vi "GetProbePlanCoordinates.vi"(8 "Use index as X coord":bool=TRUE, 9 "Probe Card Channels":i32=1) -> (0 "file path":string, 2 "OK?":bool, 3 "Array":T1(array[cluster]))   [LabVIEW 2018] (continued)
616", "Coord On/Off"=TRUE}, {"X"=617.0, "Y"=0.0, "Label"="Strip\t617", "Coord On/Off"=TRUE}, {"X"=618.0, "Y"=0.0, "Label"="Strip\t618", "Coord On/Off"=TRUE}, {"X"=619.0, "Y"=0.0, "Label"="Strip\t619", "Coord On/Off"=TRUE}, {"X"=620.0, "Y"=0.0, "Label"="Strip\t620", "Coord On/Off"=TRUE}, {"X"=621.0, "Y"=0.0, "Label"="Strip\t621", "Coord On/Off"=TRUE}, {"X"=622.0, "Y"=0.0, "Label"="Strip\t622", "Coord On/Off"=TRUE}, {"X"=623.0, "Y"=0.0, "Label"="Strip\t623", "Coord On/Off"=TRUE}, {"X"=624.0, "Y"=0.0, "Label"="Strip\t624", "Coord On/Off"=TRUE}, {"X"=625.0, "Y"=0.0, "Label"="Strip\t625", "Coord On/Off"=TRUE}, {"X"=626.0, "Y"=0.0, "Label"="Strip\t626", "Coord On/Off"=TRUE}, {"X"=627.0, "Y"=0.0, "Label"="Strip\t627", "Coord On/Off"=TRUE}, {"X"=628.0, "Y"=0.0, "Label"="Strip\t628", "Coord On/Off"=TRUE}, {"X"=629.0, "Y"=0.0, "Label"="Strip\t629", "Coord On/Off"=TRUE}, {"X"=630.0, "Y"=0.0, "Label"="Strip\t630", "Coord On/Off"=TRUE}, {"X"=631.0, "Y"=0.0, "Label"="Strip\t631", "Coord On/Off"=TRUE}, {"X"=632.0, "Y"=0.0, "Label"="Strip\t632", "Coord On/Off"=TRUE}, {"X"=633.0, "Y"=0.0, "Label"="Strip\t633", "Coord On/Off"=TRUE}, {"X"=634.0, "Y"=0.0, "Label"="Strip\t634", "Coord On/Off"=TRUE}, {"X"=635.0, "Y"=0.0, "Label"="Strip\t635", "Coord On/Off"=TRUE}, {"X"=636.0, "Y"=0.0, "Label"="Strip\t636", "Coord On/Off"=TRUE}, {"X"=637.0, "Y"=0.0, "Label"="Strip\t637", "Coord On/Off"=TRUE}, {"X"=638.0, "Y"=0.0, "Label"="Strip\t638", "Coord On/Off"=TRUE}, {"X"=639.0, "Y"=0.0, "Label"="Strip\t639", "Coord On/Off"=TRUE}, {"X"=640.0, "Y"=0.0, "Label"="Strip\t640", "Coord On/Off"=TRUE}, {"X"=641.0, "Y"=0.0, "Label"="Strip\t641", "Coord On/Off"=TRUE}, {"X"=642.0, "Y"=0.0, "Label"="Strip\t642", "Coord On/Off"=TRUE}, {"X"=643.0, "Y"=0.0, "Label"="Strip\t643", "Coord On/Off"=TRUE}, {"X"=644.0, "Y"=0.0, "Label"="Strip\t644", "Coord On/Off"=TRUE}, {"X"=645.0, "Y"=0.0, "Label"="Strip\t645", "Coord On/Off"=TRUE}, {"X"=646.0, "Y"=0.0, "Label"="Strip\t646", "Coord On/Off"=TRUE}, {"X"=647.0, "Y"=0.0, "Label"="Strip\t647", "Coord On/Off"=TRUE}, {"X"=648.0, "Y"=0.0, "Label"="Strip\t648", "Coord On/Off"=TRUE}, {"X"=649.0, "Y"=0.0, "Label"="Strip\t649", "Coord On/Off"=TRUE}, {"X"=650.0, "Y"=0.0, "Label"="Strip\t650", "Coord On/Off"=TRUE}, {"X"=651.0, "Y"=0.0, "Label"="Strip\t651", "Coord On/Off"=TRUE}, {"X"=652.0, "Y"=0.0, "Label"="Strip\t652", "Coord On/Off"=TRUE}, {"X"=653.0, "Y"=0.0, "Label"="Strip\t653", "Coord On/Off"=TRUE}, {"X"=654.0, "Y"=0.0, "Label"="Strip\t654", "Coord On/Off"=TRUE}, {"X"=655.0, "Y"=0.0, "Label"="Strip\t655", "Coord On/Off"=TRUE}, {"X"=656.0, "Y"=0.0, "Label"="Strip\t656", "Coord On/Off"=TRUE}, {"X"=657.0, "Y"=0.0, "Label"="Strip\t657", "Coord On/Off"=TRUE}, {"X"=658.0, "Y"=0.0, "Label"="Strip\t658", "Coord On/Off"=TRUE}, {"X"=659.0, "Y"=0.0, "Label"="Strip\t659", "Coord On/Off"=TRUE}, {"X"=660.0, "Y"=0.0, "Label"="Strip\t660", "Coord On/Off"=TRUE}, {"X"=661.0, "Y"=0.0, "Label"="Strip\t661", "Coord On/Off"=TRUE}, {"X"=662.0, "Y"=0.0, "Label"="Strip\t662", "Coord On/Off"=TRUE}, {"X"=663.0, "Y"=0.0, "Label"="Strip\t663", "Coord On/Off"=TRUE}, {"X"=664.0, "Y"=0.0, "Label"="Strip\t664", "Coord On/Off"=TRUE}, {"X"=665.0, "Y"=0.0, "Label"="Strip\t665", "Coord On/Off"=TRUE}, {"X"=666.0, "Y"=0.0, "Label"="Strip\t666", "Coord On/Off"=TRUE}, {"X"=667.0, "Y"=0.0, "Label"="Strip\t667", "Coord On/Off"=TRUE}, {"X"=668.0, "Y"=0.0, "Label"="Strip\t668", "Coord On/Off"=TRUE}, {"X"=669.0, "Y"=0.0, "Label"="Strip\t669", "Coord On/Off"=TRUE}, {"X"=670.0, "Y"=0.0, "Label"="Strip\t670", "Coord On/Off"=TRUE}, {"X"=671.0, "Y"=0.0, "Label"="Strip\t671", "Coord On/Off"=TRUE}, {"X"=672.0, "Y"=0.0, "Label"="Strip\t672", "Coord On/Off"=TRUE}, {"X"=673.0, "Y"=0.0, "Label"="Strip\t673", "Coord On/Off"=TRUE}, {"X"=674.0, "Y"=0.0, "Label"="Strip\t674", "Coord On/Off"=TRUE}, {"X"=675.0, "Y"=0.0, "Label"="Strip\t675", "Coord On/Off"=TRUE}, {"X"=676.0, "Y"=0.0, "Label"="Strip\t676", "Coord On/Off"=TRUE}, {"X"=677.0, "Y"=0.0, "Label"="Strip\t677", "Coord On/Off"=TRUE}, {"X"=678.0, "Y"=0.0, "Label"="Strip\t678", "Coord On/Off"=TRUE}, {"X"=679.0, "Y"=0.0, "Label"="Strip\t679", "Coord On/Off"=TRUE}, {"X"=680.0, "Y"=0.0, "Label"="Strip\t680", "Coord On/Off"=TRUE}, {"X"=681.0, "Y"=0.0, "Label"="Strip\t681", "Coord On/Off"=TRUE}, {"X"=682.0, "Y"=0.0, "Label"="Strip\t682", "Coord On/Off"=TRUE}, {"X"=683.0, "Y"=0.0, "Label"="Strip\t683", "Coord On/Off"=TRUE}, {"X"=684.0, "Y"=0.0, "Label"="Strip\t684", "Coord On/Off"=TRUE}, {"X"=685.0, "Y"=0.0, "Label"="Strip\t685", "Coord On/Off"=TRUE}, {"X"=686.0, "Y"=0.0, "Label"="Strip\t686", "Coord On/Off"=TRUE}, {"X"=687.0, "Y"=0.0, "Label"="Strip\t687", "Coord On/Off"=TRUE}, {"X"=688.0, "Y"=0.0, "Label"="Strip\t688", "Coord On/Off"=TRUE}, {"X"=689.0, "Y"=0.0, "Label"="Strip\t689", "Coord On/Off"=TRUE}, {"X"=690.0, "Y"=0.0, "Label"="Strip\t690", "Coord On/Off"=TRUE}, {"X"=691.0, "Y"=0.0, "Label"="Strip\t691", "Coord On/Off"=TRUE}, {"X"=692.0, "Y"=0.0, "Label"="Strip\t692", "Coord On/Off"=TRUE}, {"X"=693.0, "Y"=0.0, "Label"="Strip\t693", "Coord On/Off"=TRUE}, {"X"=694.0, "Y"=0.0, "Label"="Strip\t694", "Coord On/Off"=TRUE}, {"X"=695.0, "Y"=0.0, "Label"="Strip\t695", "Coord On/Off"=TRUE}, {"X"=696.0, "Y"=0.0, "Label"="Strip\t696", "Coord On/Off"=TRUE}, {"X"=697.0, "Y"=0.0, "Label"="Strip\t697", "Coord On/Off"=TRUE}, {"X"=698.0, "Y"=0.0, "Label"="Strip\t698", "Coord On/Off"=TRUE}, {"X"=699.0, "Y"=0.0, "Label"="Strip\t699", "Coord On/Off"=TRUE}, {"X"=700.0, "Y"=0.0, "Label"="Strip\t700", "Coord On/Off"=TRUE}, {"X"=701.0, "Y"=0.0, "Label"="Strip\t701", "Coord On/Off"=TRUE}, {"X"=702.0, "Y"=0.0, "Label"="Strip\t702", "Coord On/Off"=TRUE}, {"X"=703.0, "Y"=0.0, "Label"="Strip\t703", "Coord On/Off"=TRUE}, {"X"=704.0, "Y"=0.0, "Label"="Strip\t704", "Coord On/Off"=TRUE}, {"X"=705.0, "Y"=0.0, "Label"="Strip\t705", "Coord On/Off"=TRUE}, {"X"=706.0, "Y"=0.0, "Label"="Strip\t706", "Coord On/Off"=TRUE}, {"X"=707.0, "Y"=0.0, "Label"="Strip\t707", "Coord On/Off"=TRUE}, {"X"=708.0, "Y"=0.0, "Label"="Strip\t708", "Coord On/Off"=TRUE}, {"X"=709.0, "Y"=0.0, "Label"="Strip\t709", "Coord On/Off"=TRUE}, {"X"=710.0, "Y"=0.0, "Label"="Strip\t710", "Coord On/Off"=TRUE}, {"X"=711.0, "Y"=0.0, "Label"="Strip\t711", "Coord On/Off"=TRUE}, {"X"=712.0, "Y"=0.0, "Label"="Strip\t712", "Coord On/Off"=TRUE}, {"X"=713.0, "Y"=0.0, "Label"="Strip\t713", "Coord On/Off"=TRUE}, {"X"=714.0, "Y"=0.0, "Label"="Strip\t714", "Coord On/Off"=TRUE}, {"X"=715.0, "Y"=0.0, "Label"="Strip\t715", "Coord On/Off"=TRUE}, {"X"=716.0, "Y"=0.0, "Label"="Strip\t716", "Coord On/Off"=TRUE}, {"X"=717.0, "Y"=0.0, "Label"="Strip\t717", "Coord On/Off"=TRUE}, {"X"=718.0, "Y"=0.0, "Label"="Strip\t718", "Coord On/Off"=TRUE}, {"X"=719.0, "Y"=0.0, "Label"="Strip\t719", "Coord On/Off"=TRUE}, {"X"=720.0, "Y"=0.0, "Label"="Strip\t720", "Coord On/Off"=TRUE}, {"X"=721.0, "Y"=0.0, "Label"="Strip\t721", "Coord On/Off"=TRUE}, {"X"=722.0, "Y"=0.0, "Label"="Strip\t722", "Coord On/Off"=TRUE}, {"X"=723.0, "Y"=0.0, "Label"="Strip\t723", "Coord On/Off"=TRUE}, {"X"=724.0, "Y"=0.0, "Label"="Strip\t724", "Coord On/Off"=TRUE}, {"X"=725.0, "Y"=0.0, "Label"="Strip\t725", "Coord On/Off"=TRUE}, {"X"=726.0, "Y"=0.0, "Label"="Strip\t726", "Coord On/Off"=TRUE}, {"X"=727.0, "Y"=0.0, "Label"="Strip\t727", "Coord On/Off"=TRUE}, {"X"=728.0, "Y"=0.0, "Label"="Strip\t728", "Coord On/Off"=TRUE}, {"X"=729.0, "Y"=0.0, "Label"="Strip\t729", "Coord On/Off"=TRUE}, {"X"=730.0, "Y"=0.0, "Label"="Strip\t730", "Coord On/Off"=TRUE}, {"X"=731.0, "Y"=0.0, "Label"="Strip\t731", "Coord On/Off"=TRUE}, {"X"=732.0, "Y"=0.0, "Label"="Strip\t732", "Coord On/Off"=TRUE}, {"X"=733.0, "Y"=0.0, "Label"="Strip\t733", "Coord On/Off"=TRUE}, {"X"=734.0, "Y"=0.0, "Label"="Strip\t734", "Coord On/Off"=TRUE}, {"X"=735.0, "Y"=0.0, "Label"="Strip\t735", "Coord On/Off"=TRUE}, {"X"=736.0, "Y"=0.0, "Label"="Strip\t736", "Coord On/Off"=TRUE}, {"X"=737.0, "Y"=0.0, "Label"="Strip\t737", "Coord On/Off"=TRUE}, {"X"=738.0, "Y"=0.0, "Label"="Strip\t738", "Coord On/Off"=TRUE}, {"X"=739.0, "Y"=0.0, "Label"="Strip\t739", "Coord On/Off"=TRUE}, {"X"=740.0, "Y"=0.0, "Label"="Strip\t740", "Coord On/Off"=TRUE}, {"X"=741.0, "Y"=0.0, "Label"="Strip\t741", "Coord On/Off"=TRUE}, {"X"=742.0, "Y"=0.0, "Label"="Strip\t742", "Coord On/Off"=TRUE}, {"X"=743.0, "Y"=0.0, "Label"="Strip\t743", "Coord On/Off"=TRUE}, {"X"=744.0, "Y"=0.0, "Label"="Strip\t744", "Coord On/Off"=TRUE}, {"X"=745.0, "Y"=0.0, "Label"="Strip\t745", "Coord On/Off"=TRUE}, {"X"=746.0, "Y"=0.0, "Label"="Strip\t746", "Coord On/Off"=TRUE}, {"X"=747.0, "Y"=0.0, "Label"="Strip\t747", "Coord On/Off"=TRUE}, {"X"=748.0, "Y"=0.0, "Label"="Strip\t748", "Coord On/Off"=TRUE}, {"X"=749.0, "Y"=0.0, "Label"="Strip\t749", "Coord On/Off"=TRUE}, {"X"=750.0, "Y"=0.0, "Label"="Strip\t750", "Coord On/Off"=TRUE}, {"X"=751.0, "Y"=0.0, "Label"="Strip\t751", "Coord On/Off"=TRUE}, {"X"=752.0, "Y"=0.0, "Label"="Strip\t752", "Coord On/Off"=TRUE}, {"X"=753.0, "Y"=0.0, "Label"="Strip\t753", "Coord On/Off"=TRUE}, {"X"=754.0, "Y"=0.0, "Label"="Strip\t754", "Coord On/Off"=TRUE}, {"X"=755.0, "Y"=0.0, "Label"="Strip\t755", "Coord On/Off"=TRUE}, {"X"=756.0, "Y"=0.0, "Label"="Strip\t756", "Coord On/Off"=TRUE}, {"X"=757.0, "Y"=0.0, "Label"="Strip\t757", "Coord On/Off"=TRUE}, {"X"=758.0, "Y"=0.0, "Label"="Strip\t758", "Coord On/Off"=TRUE}, {"X"=759.0, "Y"=0.0, "Label"="Strip\t759", "Coord On/Off"=TRUE}, {"X"=760.0, "Y"=0.0, "Label"="Strip\t760", "Coord On/Off"=TRUE}, {"X"=761.0, "Y"=0.0, "Label"="Strip\t761", "Coord On/Off"=TRUE}, {"X"=762.0, "Y"=0.0, "Label"="Strip\t762", "Coord On/Off"=TRUE}, {"X"=763.0, "Y"=0.0, "Label"="Strip\t763", "Coord On/Off"=TRUE}, {"X"=764.0, "Y"=0.0, "Label"="Strip\t764", "Coord On/Off"=TRUE}, {"X"=765.0, "Y"=0.0, "Label"="Strip\t765", "Coord On/Off"=TRUE}, {"X"=766.0, "Y"=0.0, "Label"="Strip\t766", "Coord On/Off"=TRUE}, {"X"=767.0, "Y"=0.0, "Label"="Strip\t767", "Coord On/Off"=TRUE}, {"X"=768.0, "Y"=0.0, "Label"="Strip\t768", "Coord On/Off"=TRUE}, {"X"=769.0, "Y"=0.0, "Label"="Strip\t769", "Coord On/Off"=TRUE}, {"X"=770.0, "Y"=0.0, "Label"="Strip\t770", "Coord On/Off"=TRUE}, {"X"=771.0, "Y"=0.0, "Label"="Strip\t771", "Coord On/Off"=TRUE}, {"X"=772.0, "Y"=0.0, "Label"="Strip\t772", "Coord On/Off"=TRUE}, {"X"=773.0, "Y"=0.0, "Label"="Strip\t773", "Coord On/Off"=TRUE}, {"X"=774.0, "Y"=0.0, "Label"="Strip\t774", "Coord On/Off"=TRUE}, {"X"=775.0, "Y"=0.0, "Label"="Strip\t775", "Coord On/Off"=TRUE}, {"X"=776.0, "Y"=0.0, "Label"="Strip\t776", "Coord On/Off"=TRUE}, {"X"=777.0, "Y"=0.0, "Label"="Strip\t777", "Coord On/Off"=TRUE}, {"X"=778.0, "Y"=0.0, "Label"="Strip\t778", "Coord On/Off"=TRUE}, {"X"=779.0, "Y"=0.0, "Label"="Strip\t779", "Coord On/Off"=TRUE}, {"X"=780.0, "Y"=0.0, "Label"="Strip\t780", "Coord On/Off"=TRUE}, {"X"=781.0, "Y"=0.0, "Label"="Strip\t781", "Coord On/Off"=TRUE}, {"X"=782.0, "Y"=0.0, "Label"="Strip\t782", "Coord On/Off"=TRUE}, {"X"=783.0, "Y"=0.0, "Label"="Strip\t783", "Coord On/Off"=TRUE}, {"X"=784.0, "Y"=0.0, "Label"="Strip\t784", "Coord On/Off"=TRUE}, {"X"=785.0, "Y"=0.0, "Label"="Strip\t785", "Coord On/Off"=TRUE}, {"X"=786.0, "Y"=0.0, "Label"="Strip\t786", "Coord On/Off"=TRUE}, {"X"=787.0, "Y"=0.0, "Label"="Strip\t787", "Coord On/Off"=TRUE}, {"X"=788.0, "Y"=0.0, "Label"="Strip\t788", "Coord On/Off"=TRUE}, {"X"=789.0, "Y"=0.0, "Label"="Strip\t789", "Coord On/Off"=TRUE}, {"X"=790.0, "Y"=0.0, "Label"="Strip\t790", "Coord On/Off"=TRUE}, {"X"=791.0, "Y"=0.0, "Label"="Strip\t791", "Coord On/Off"=TRUE}, {"X"=792.0, "Y"=0.0, "Label"="Strip\t792", "Coord On/Off"=TRUE}, {"X"=793.0, "Y"=0.0, "Label"="Strip\t793", "Coord On/Off"=TRUE}, {"X"=794.0, "Y"=0.0, "Label"="Strip\t794", "Coord On/Off"=TRUE}, {"X"=795.0, "Y"=0.0, "Label"="Strip\t795", "Coord On/Off"=TRUE}, {"X"=796.0, "Y"=0.0, "Label"="Strip\t796", "Coord On/Off"=TRUE}, {"X"=797.0, "Y"=0.0, "Label"="Strip\t797", "Coord On/Off"=TRUE}, {"X"=798.0, "Y"=0.0, "Label"="Strip\t798", "Coord On/Off"=TRUE}, {"X"=799.0, "Y"=0.0, "Label"="Strip\t799", "Coord On/Off"=TRUE}, {"X"=800.0, "Y"=0.0, "Label"="Strip\t800", "Coord On/Off"=TRUE}, {"X"=801.0, "Y"=0.0, "Label"="Strip\t801", "Coord On/Off"=TRUE}, {"X"=802.0, "Y"=0.0, "Label"="Strip\t802", "Coord On/Off"=TRUE}, {"X"=803.0, "Y"=0.0, "Label"="Strip\t803", "Coord On/Off"=TRUE}, {"X"=804.0, "Y"=0.0, "Label"="Strip\t804", "Coord On/Off"=TRUE}, {"X"=805.0, "Y"=0.0, "Label"="Strip\t805", "Coord On/Off"=TRUE}, {"X"=806.0, "Y"=0.0, "Label"="Strip\t806", "Coord On/Off"=TRUE}, {"X"=807.0, "Y"=0.0, "Label"="Strip\t807", "Coord On/Off"=TRUE}, {"X"=808.0, "Y"=0.0, "Label"="Strip\t808", "Coord On/Off"=TRUE}, {"X"=809.0, "Y"=0.0, "Label"="Strip\t809", "Coord On/Off"=TRUE}, {"X"=810.0, "Y"=0.0, "Label"="Strip\t810", "Coord On/Off"=TRUE}, {"X"=811.0, "Y"=0.0, "Label"="Strip\t811", "Coord On/Off"=TRUE}, {"X"=812.0, "Y"=0.0, "Label"="Strip\t812", "Coord On/Off"=TRUE}, {"X"=813.0, "Y"=0.0, "Label"="Strip\t813", "Coord On/Off"=TRUE}, {"X"=814.0, "Y"=0.0, "Label"="Strip\t814", "Coord On/Off"=TRUE}, {"X"=815.0, "Y"=0.0, "Label"="Strip\t815", "Coord On/Off"=TRUE}, {"X"=816.0, "Y"=0.0, "Label"="Strip\t816", "Coord On/Off"=TRUE}, {"X"=817.0, "Y"=0.0, "Label"="Strip\t817", "Coord On/Off"=TRUE}, {"X"=818.0, "Y"=0.0, "Label"="Strip\t818", "Coord On/Off"=TRUE}, {"X"=819.0, "Y"=0.0, "Label"="Strip\t819", "Coord On/Off"=TRUE}, {"X"=820.0, "Y"=0.0, "Label"="Strip\t820", "Coord On/Off"=TRUE}, {"X"=821.0, "Y"=0.0, "Label"="Strip\t821", "Coord On/Off"=TRUE}, {"X"=822.0, "Y"=0.0, "Label"="Strip\t822", "Coord On/Off"=TRUE}, {"X"=823.0, "Y"=0.0, "Label"="Strip\t823", "Coord On/Off"=TRUE}, {"X"=824.0, "Y"=0.0, "Label"="Strip\t824", "Coord On/Off"=TRUE}, {"X"=825.0, "Y"=0.0, "Label"="Strip\t825", "Coord On/Off"=TRUE}, {"X"=826.0, "Y"=0.0, "Label"="Strip\t826", "Coord On/Off"=TRUE}, {"X"=827.0, "Y"=0.0, "Label"="Strip\t827", "Coord On/Off"=TRUE}, {"X"=828.0, "Y"=0.0, "Label"="Strip\t828", "Coord On/Off"=TRUE}, {"X"=829.0, "Y"=0.0, "Label"="Strip\t829", "Coord On/Off"=TRUE}, {"X"=830.0, "Y"=0.0, "Label"="Strip\t830", "Coord On/Off"=TRUE}, {"X"=831.0, "Y"=0.0, "Label"="Strip\t831", "Coord On/Off"=TRUE}, {"X"=832.0, "Y"=0.0, "Label"="Strip\t832", "Coord On/Off"=TRUE}, {"X"=833.0, "Y"=0.0, "Label"="Strip\t833", "Coord On/Off"=TRUE}, {"X"=834.0, "Y"=0.0, "Label"="Strip\t834", "Coord On/Off"=TRUE}, {"X"=835.0, "Y"=0.0, "Label"="Strip\t835", "Coord On/Off"=TRUE}, {"X"=836.0, "Y"=0.0, "Label"="Strip\t836", "Coord On/Off"=TRUE}, {"X"=837.0, "Y"=0.0, "Label"="Strip\t837", "Coord On/Off"=TRUE}, {"X"=838.0, "Y"=0.0, "Label"="Strip\t838", "Coord On/Off"=TRUE}, {"X"=839.0, "Y"=0.0, "Label"="Strip\t839", "Coord On/Off"=TRUE}, {"X"=840.0, "Y"=0.0, "Label"="Strip\t840", "Coord On/Off"=TRUE}, {"X"=841.0, "Y"=0.0, "Label"="Strip\t841", "Coord On/Off"=TRUE}, {"X"=842.0, "Y"=0.0, "Label"="Strip\t842", "Coord On/Off"=TRUE}, {"X"=843.0, "Y"=0.0, "Label"="Strip\t843", "Coord On/Off"=TRUE}, {"X"=844.0, "Y"=0.0, "Label"="Strip\t844", "Coord On/Off"=TRUE}, {"X"=845.0, "Y"=0.0, "Label"="Strip\t845", "Coord On/Off"=TRUE}, {"X"=846.0, "Y"=0.0, "Label"="Strip\t846", "Coord On/Off"=TRUE}, {"X"=847.0, "Y"=0.0, "Label"="Strip\t847", "Coord On/Off"=TRUE}, {"X"=848.0, "Y"=0.0, "Label"="Strip\t848", "Coord On/Off"=TRUE}, {"X"=849.0, "Y"=0.0, "Label"="Strip\t849", "Coord On/Off"=TRUE}, {"X"=850.0, "Y"=0.0, "Label"="Strip\t850", "Coord On/Off"=TRUE}, {"X"=851.0, "Y"=0.0, "Label"="Strip\t851", "Coord On/Off"=TRUE}, {"X"=852.0, "Y"=0.0, "Label"="Strip\t852", "Coord On/Off"=TRUE}, {"X"=853.0, "Y"=0.0, "Label"="Strip\t853", "Coord On/Off"=TRUE}, {"X"=854.0, "Y"=0.0, "Label"="Strip\t854", "Coord On/Off"=TRUE}, {"X"=855.0, "Y"=0.0, "Label"="Strip\t855", "Coord On/Off"=TRUE}, {"X"=856.0, "Y"=0.0, "Label"="Strip\t856", "Coord On/Off"=TRUE}, {"X"=857.0, "Y"=0.0, "Label"="Strip\t857", "Coord On/Off"=TRUE}, {"X"=858.0, "Y"=0.0, "Label"="Strip\t858", "Coord On/Off"=TRUE}, {"X"=859.0, "Y"=0.0, "Label"="Strip\t859", "Coord On/Off"=TRUE}, {"X"=860.0, "Y"=0.0, "Label"="Strip\t860", "Coord On/Off"=TRUE}, {"X"=861.0, "Y"=0.0, "Label"="Strip\t861", "Coord On/Off"=TRUE}, {"X"=862.0, "Y"=0.0, "Label"="Strip\t862", "Coord On/Off"=TRUE}, {"X"=863.0, "Y"=0.0, "Label"="Strip\t863", "Coord On/Off"=TRUE}, {"X"=864.0, "Y"=0.0, "Label"="Strip\t864", "Coord On/Off"=TRUE}, {"X"=865.0, "Y"=0.0, "Label"="Strip\t865", "Coord On/Off"=TRUE}, {"X"=866.0, "Y"=0.0, "Label"="Strip\t866", "Coord On/Off"=TRUE}, {"X"=867.0, "Y"=0.0, "Label"="Strip\t867", "Coord On/Off"=TRUE}, {"X"=868.0, "Y"=0.0, "Label"="Strip\t868", "Coord On/Off"=TRUE}, {"X"=869.0, "Y"=0.0, "Label"="Strip\t869", "Coord On/Off"=TRUE}, {"X"=870.0, "Y"=0.0, "Label"="Strip\t870", "Coord On/Off"=TRUE}, {"X"=871.0, "Y"=0.0, "Label"="Strip\t871", "Coord On/Off"=TRUE}, {"X"=872.0, "Y"=0.0, "Label"="Strip\t872", "Coord On/Off"=TRUE}, {"X"=873.0, "Y"=0.0, "Label"="Strip\t873", "Coord On/Off"=TRUE}, {"X"=874.0, "Y"=0.0, "Label"="Strip\t874", "Coord On/Off"=TRUE}, {"X"=875.0, "Y"=0.0, "Label"="Strip\t875", "Coord On/Off"=TRUE}, {"X"=876.0, "Y"=0.0, "Label"="Strip\t876", "Coord On/Off"=TRUE}, {"X"=877.0, "Y"=0.0, "Label"="Strip\t877", "Coord On/Off"=TRUE}, {"X"=878.0, "Y"=0.0, "Label"="Strip\t878", "Coord On/Off"=TRUE}, {"X"=879.0, "Y"=0.0, "Label"="Strip\t879", "Coord On/Off"=TRUE}, {"X"=880.0, "Y"=0.0, "Label"="Strip\t880", "Coord On/Off"=TRUE}, {"X"=881.0, "Y"=0.0, "Label"="Strip\t881", "Coord On/Off"=TRUE}, {"X"=882.0, "Y"=0.0, "Label"="Strip\t882", "Coord On/Off"=TRUE}, {"X"=883.0, "Y"=0.0, "Label"="Strip\t883", "Coord On/Off"=TRUE}, {"X"=884.0, "Y"=0.0, "Label"="Strip\t884", "Coord On/Off"=TRUE}, {"X"=885.0, "Y"=0.0, "Label"="Strip\t885", "Coord On/Off"=TRUE}, {"X"=886.0, "Y"=0.0, "Label"="Strip\t886", "Coord On/Off"=TRUE}, {"X"=887.0, "Y"=0.0, "Label"="Strip\t887", "Coord On/Off"=TRUE}, {"X"=888.0, "Y"=0.0, "Label"="Strip\t888", "Coord On/Off"=TRUE}, {"X"=889.0, "Y"=0.0, "Label"="Strip\t889", "Coord On/Off"=TRUE}, {"X"=890.0, "Y"=0.0, "Label"="Strip\t890", "Coord On/Off"=TRUE}, {"X"=891.0, "Y"=0.0, "Label"="Strip\t891", "Coord On/Off"=TRUE}, {"X"=892.0, "Y"=0.0, "Label"="Strip\t892", "Coord On/Off"=TRUE}, {"X"=893.0, "Y"=0.0, "Label"="Strip\t893", "Coord On/Off"=TRUE}, {"X"=894.0, "Y"=0.0, "Label"="Strip\t894", "Coord On/Off"=TRUE}, {"X"=895.0, "Y"=0.0, "Label"="Strip\t895", "Coord On/Off"=TRUE}, {"X"=896.0, "Y"=0.0, "Label"="Strip\t896", "Coord On/Off"=TRUE}, {"X"=897.0, "Y"=0.0, "Label"="Strip\t897", "Coord On/Off"=TRUE}, {"X"=898.0, "Y"=0.0, "Label"="Strip\t898", "Coord On/Off"=TRUE}, {"X"=899.0, "Y"=0.0, "Label"="Strip\t899", "Coord On/Off"=TRUE}, {"X"=900.0, "Y"=0.0, "Label"="Strip\t900", "Coord On/Off"=TRUE}, {"X"=901.0, "Y"=0.0, "Label"="Strip\t901", "Coord On/Off"=TRUE}, {"X"=902.0, "Y"=0.0, "Label"="Strip\t902", "Coord On/Off"=TRUE}, {"X"=903.0, "Y"=0.0, "Label"="Strip\t903", "Coord On/Off"=TRUE}, {"X"=904.0, "Y"=0.0, "Label"="Strip\t904", "Coord On/Off"=TRUE}, {"X"=905.0, "Y"=0.0, "Label"="Strip\t905", "Coord On/Off"=TRUE}, {"X"=906.0, "Y"=0.0, "Label"="Strip\t906", "Coord On/Off"=TRUE}, {"X"=907.0, "Y"=0.0, "Label"="Strip\t907", "Coord On/Off"=TRUE}, {"X"=908.0, "Y"=0.0, "Label"="Strip\t908", "Coord On/Off"=TRUE}, {"X"=909.0, "Y"=0.0, "Label"="Strip\t909", "Coord On/Off"=TRUE}, {"X"=910.0, "Y"=0.0, "Label"="Strip\t910", "Coord On/Off"=TRUE}, {"X"=911.0, "Y"=0.0, "Label"="Strip\t911", "Coord On/Off"=TRUE}, {"X"=912.0, "Y"=0.0, "Label"="Strip\t912", "Coord On/Off"=TRUE}, {"X"=913.0, "Y"=0.0, "Label"="Strip\t913", "Coord On/Off"=TRUE}, {"X"=914.0, "Y"=0.0, "Label"="Strip\t914", "Coord On/Off"=TRUE}, {"X"=915.0, "Y"=0.0, "Label"="Strip\t915", "Coord On/Off"=TRUE}, {"X"=916.0, "Y"=0.0, "Label"="Strip\t916", "Coord On/Off"=TRUE}, {"X"=917.0, "Y"=0.0, "Label"="Strip\t917", "Coord On/Off"=TRUE}, {"X"=918.0, "Y"=0.0, "Label"="Strip\t918", "Coord On/Off"=TRUE}, {"X"=919.0, "Y"=0.0, "Label"="Strip\t919", "Coord On/Off"=TRUE}, {"X"=920.0, "Y"=0.0, "Label"="Strip\t920", "Coord On/Off"=TRUE}, {"X"=921.0, "Y"=0.0, "Label"="Strip\t921", "Coord On/Off"=TRUE}, {"X"=922.0, "Y"=0.0, "Label"="Strip\t922", "Coord On/Off"=TRUE}, {"X"=923.0, "Y"=0.0, "Label"="Strip\t923", "Coord On/Off"=TRUE}, {"X"=924.0, "Y"=0.0, "Label"="Strip\t924", "Coord On/Off"=TRUE}, {"X"=925.0, "Y"=0.0, "Label"="Strip\t925", "Coord On/Off"=TRUE}, {"X"=926.0, "Y"=0.0, "Label"="Strip\t926", "Coord On/Off"=TRUE}, {"X"=927.0, "Y"=0.0, "Label"="Strip\t927", "Coord On/Off"=TRUE}, {"X"=928.0, "Y"=0.0, "Label"="Strip\t928", "Coord On/Off"=TRUE}, {"X"=929.0, "Y"=0.0, "Label"="Strip\t929", "Coord On/Off"=TRUE}, {"X"=930.0, "Y"=0.0, "Label"="Strip\t930", "Coord On/Off"=TRUE}, {"X"=931.0, "Y"=0.0, "Label"="Strip\t931", "Coord On/Off"=TRUE}, {"X"=932.0, "Y"=0.0, "Label"="Strip\t932", "Coord On/Off"=TRUE}, {"X"=933.0, "Y"=0.0, "Label"="Strip\t933", "Coord On/Off"=TRUE}, {"X"=934.0, "Y"=0.0, "Label"="Strip\t934", "Coord On/Off"=TRUE}, {"X"=935.0, "Y"=0.0, "Label"="Strip\t935", "Coord On/Off"=TRUE}, {"X"=936.0, "Y"=0.0, "Label"="Strip\t936", "Coord On/Off"=TRUE}, {"X"=937.0, "Y"=0.0, "Label"="Strip\t937", "Coord On/Off"=TRUE}, {"X"=938.0, "Y"=0.0, "Label"="Strip\t938", "Coord On/Off"=TRUE}, {"X"=939.0, "Y"=0.0, "Label"="Strip\t939", "Coord On/Off"=TRUE}, {"X"=940.0, "Y"=0.0, "Label"="Strip\t940", "Coord On/Off"=TRUE}, {"X"=941.0, "Y"=0.0, "Label"="Strip\t941", "Coord On/Off"=TRUE}, {"X"=942.0, "Y"=0.0, "Label"="Strip\t942", "Coord On/Off"=TRUE}, {"X"=943.0, "Y"=0.0, "Label"="Strip\t943", "Coord On/Off"=TRUE}, {"X"=944.0, "Y"=0.0, "Label"="Strip\t944", "Coord On/Off"=TRUE}, {"X"=945.0, "Y"=0.0, "Label"="Strip\t945", "Coord On/Off"=TRUE}, {"X"=946.0, "Y"=0.0, "Label"="Strip\t946", "Coord On/Off"=TRUE}, {"X"=947.0, "Y"=0.0, "Label"="Strip\t947", "Coord On/Off"=TRUE}, {"X"=948.0, "Y"=0.0, "Label"="Strip\t948", "Coord On/Off"=TRUE}, {"X"=949.0, "Y"=0.0, "Label"="Strip\t949", "Coord On/Off"=TRUE}, {"X"=950.0, "Y"=0.0, "Label"="Strip\t950", "Coord On/Off"=TRUE}, {"X"=951.0, "Y"=0.0, "Label"="Strip\t951", "Coord On/Off"=TRUE}, {"X"=952.0, "Y"=0.0, "Label"="Strip\t952", "Coord On/Off"=TRUE}, {"X"=953.0, "Y"=0.0, "Label"="Strip\t953", "Coord On/Off"=TRUE}, {"X"=954.0, "Y"=0.0, "Label"="Strip\t954", "Coord On/Off"=TRUE}, {"X"=955.0, "Y"=0.0, "Label"="Strip\t955", "Coord On/Off"=TRUE}, {"X"=956.0, "Y"=0.0, "Label"="Strip\t956", "Coord On/Off"=TRUE}, {"X"=957.0, "Y"=0.0, "Label"="Strip\t957", "Coord On/Off"=TRUE}, {"X"=958.0, "Y"=0.0, "Label"="Strip\t958", "Coord On/Off"=TRUE}, {"X"=959.0, "Y"=0.0, "Label"="Strip\t959", "Coord On/Off"=TRUE}, {"X"=960.0, "Y"=0.0, "Label"="Strip\t960", "Coord On/Off"=TRUE}, {"X"=961.0, "Y"=0.0, "Label"="Strip\t961", "Coord On/Off"=TRUE}, {"X"=962.0, "Y"=0.0, "Label"="Strip\t962", "Coord On/Off"=TRUE}, {"X"=963.0, "Y"=0.0, "Label"="Strip\t963", "Coord On/Off"=TRUE}, {"X"=964.0, "Y"=0.0, "Label"="Strip\t964", "Coord On/Off"=TRUE}, {"X"=965.0, "Y"=0.0, "Label"="Strip\t965", "Coord On/Off"=TRUE}, {"X"=966.0, "Y"=0.0, "Label"="Strip\t966", "Coord On/Off"=TRUE}, {"X"=967.0, "Y"=0.0, "Label"="Strip\t967", "Coord On/Off"=TRUE}, {"X"=968.0, "Y"=0.0, "Label"="Strip\t968", "Coord On/Off"=TRUE}, {"X"=969.0, "Y"=0.0, "Label"="Strip\t969", "Coord On/Off"=TRUE}, {"X"=970.0, "Y"=0.0, "Label"="Strip\t970", "Coord On/Off"=TRUE}, {"X"=971.0, "Y"=0.0, "Label"="Strip\t971", "Coord On/Off"=TRUE}, {"X"=972.0, "Y"=0.0, "Label"="Strip\t972", "Coord On/Off"=TRUE}, {"X"=973.0, "Y"=0.0, "Label"="Strip\t973", "Coord On/Off"=TRUE}, {"X"=974.0, "Y"=0.0, "Label"="Strip\t974", "Coord On/Off"=TRUE}, {"X"=975.0, "Y"=0.0, "Label"="Strip\t975", "Coord On/Off"=TRUE}, {"X"=976.0, "Y"=0.0, "Label"="Strip\t976", "Coord On/Off"=TRUE}, {"X"=977.0, "Y"=0.0, "Label"="Strip\t977", "Coord On/Off"=TRUE}, {"X"=978.0, "Y"=0.0, "Label"="Strip\t978", "Coord On/Off"=TRUE}, {"X"=979.0, "Y"=0.0, "Label"="Strip\t979", "Coord On/Off"=TRUE}, {"X"=980.0, "Y"=0.0, "Label"="Strip\t980", "Coord On/Off"=TRUE}, {"X"=981.0, "Y"=0.0, "Label"="Strip\t981", "Coord On/Off"=TRUE}, {"X"=982.0, "Y"=0.0, "Label"="Strip\t982", "Coord On/Off"=TRUE}, {"X"=983.0, "Y"=0.0, "Label"="Strip\t983", "Coord On/Off"=TRUE}, {"X"=984.0, "Y"=0.0, "Label"="Strip\t984", "Coord On/Off"=TRUE}, {"X"=985.0, "Y"=0.0, "Label"="Strip\t985", "Coord On/Off"=TRUE}, {"X"=986.0, "Y"=0.0, "Label"="Strip\t986", "Coord On/Off"=TRUE}, {"X"=987.0, "Y"=0.0, "Label"="Strip\t987", "Coord On/Off"=TRUE}, {"X"=988.0, "Y"=0.0, "Label"="Strip\t988", "Coord On/Off"=TRUE}, {"X"=989.0, "Y"=0.0, "Label"="Strip\t989", "Coord On/Off"=TRUE}, {"X"=990.0, "Y"=0.0, "Label"="Strip\t990", "Coord On/Off"=TRUE}, {"X"=991.0, "Y"=0.0, "Label"="Strip\t991", "Coord On/Off"=TRUE}, {"X"=992.0, "Y"=0.0, "Label"="Strip\t992", "Coord On/Off"=TRUE}, {"X"=993.0, "Y"=0.0, "Label"="Strip\t993", "Coord On/Off"=TRUE}, {"X"=994.0, "Y"=0.0, "Label"="Strip\t994", "Coord On/Off"=TRUE}, {"X"=995.0, "Y"=0.0, "Label"="Strip\t995", "Coord On/Off"=TRUE}, {"X"=996.0, "Y"=0.0, "Label"="Strip\t996", "Coord On/Off"=TRUE}, {"X"=997.0, "Y"=0.0, "Label"="Strip\t997", "Coord On/Off"=TRUE}, {"X"=998.0, "Y"=0.0, "Label"="Strip\t998", "Coord On/Off"=TRUE}, {"X"=999.0, "Y"=0.0, "Label"="Strip\t999", "Coord On/Off"=TRUE}, {"X"=1000.0, "Y"=0.0, "Label"="Strip\t1000", "Coord On/Off"=TRUE}, {"X"=1001.0, "Y"=0.0, "Label"="Strip\t1001", "Coord On/Off"=TRUE}, {"X"=1002.0, "Y"=0.0, "Label"="Strip\t1002", "Coord On/Off"=TRUE}, {"X"=1003.0, "Y"=0.0, "Label"="Strip\t1003", "Coord On/Off"=TRUE}, {"X"=1004.0, "Y"=0.0, "Label"="Strip\t1004", "Coord On/Off"=TRUE}, {"X"=1005.0, "Y"=0.0, "Label"="Strip\t1005", "Coord On/Off"=TRUE}, {"X"=1006.0, "Y"=0.0, "Label"="Strip\t1006", "Coord On/Off"=TRUE}, {"X"=1007.0, "Y"=0.0, "Label"="Strip\t1007", "Coord On/Off"=TRUE}, {"X"=1008.0, "Y"=0.0, "Label"="Strip\t1008", "Coord On/Off"=TRUE}, {"X"=1009.0, "Y"=0.0, "Label"="Strip\t1009", "Coord On/Off"=TRUE}, {"X"=1010.0, "Y"=0.0, "Label"="Strip\t1010", "Coord On/Off"=TRUE}, {"X"=1011.0, "Y"=0.0, "Label"="Strip\t1011", "Coord On/Off"=TRUE}, {"X"=1012.0, "Y"=0.0, "Label"="Strip\t1012", "Coord On/Off"=TRUE}, {"X"=1013.0, "Y"=0.0, "Label"="Strip\t1013", "Coord On/Off"=TRUE}, {"X"=1014.0, "Y"=0.0, "Label"="Strip\t1014", "Coord On/Off"=TRUE}, {"X"=1015.0, "Y"=0.0, "Label"="Strip\t1015", "Coord On/Off"=TRUE}, {"X"=1016.0, "Y"=0.0, "Label"="Strip\t1016", "Coord On/Off"=TRUE}, {"X"=1017.0, "Y"=0.0, "Label"="Strip\t1017", "Coord On/Off"=TRUE}, {"X"=1018.0, "Y"=0.0, "Label"="Strip\t1018", "Coord On/Off"=TRUE}, {"X"=1019.0, "Y"=0.0, "Label"="Strip\t1019", "Coord On/Off"=TRUE}, {"X"=1020.0, "Y"=0.0, "Label"="Strip\t1020", "Coord On/Off"=TRUE}, {"X"=1021.0, "Y"=0.0, "Label"="Strip\t1021", "Coord On/Off"=TRUE}, {"X"=1022.0, "Y"=0.0, "Label"="Strip\t1022", "Coord On/Off"=TRUE}, {"X"=1023.0, "Y"=0.0, "Label"="Strip\t1023", "Coord On/Off"=TRUE}, {"X"=1024.0, "Y"=0.0, "Label"="Strip\t1024", "Coord On/Off"=TRUE}, {"X"=1025.0, "Y"=0.0, "Label"="Strip\t1025", "Coord On/Off"=TRUE}, {"X"=1026.0, "Y"=0.0, "Label"="Strip\t1026", "Coord On/Off"=TRUE}, {"X"=1027.0, "Y"=0.0, "Label"="Strip\t1027", "Coord On/Off"=TRUE}, {"X"=1028.0, "Y"=0.0, "Label"="Strip\t1028", "Coord On/Off"=TRUE}, {"X"=1029.0, "Y"=0.0, "Label"="Strip\t1029", "Coord On/Off"=TRUE}, {"X"=1030.0, "Y"=0.0, "Label"="Strip\t1030", "Coord On/Off"=TRUE}, {"X"=1031.0, "Y"=0.0, "Label"="Strip\t1031", "Coord On/Off"=TRUE}, {"X"=1032.0, "Y"=0.0, "Label"="Strip\t1032", "Coord On/Off"=TRUE}, {"X"=1033.0, "Y"=0.0, "Label"="Strip\t1033", "Coord On/Off"=TRUE}, {"X"=1034.0, "Y"=0.0, "Label"="Strip\t1034", "Coord On/Off"=TRUE}, {"X"=1035.0, "Y"=0.0, "Label"="Strip\t1035", "Coord On/Off"=TRUE}, {"X"=1036.0, "Y"=0.0, "Label"="Strip\t1036", "Coord On/Off"=TRUE}, {"X"=1037.0, "Y"=0.0, "Label"="Strip\t1037", "Coord On/Off"=TRUE}, {"X"=1038.0, "Y"=0.0, "Label"="Strip\t1038", "Coord On/Off"=TRUE}, {"X"=1039.0, "Y"=0.0, "Label"="Strip\t1039", "Coord On/Off"=TRUE}, {"X"=1040.0, "Y"=0.0, "Label"="Strip\t1040", "Coord On/Off"=TRUE}, {"X"=1041.0, "Y"=0.0, "Label"="Strip\t1041", "Coord On/Off"=TRUE}, {"X"=1042.0, "Y"=0.0, "Label"="Strip\t1042", "Coord On/Off"=TRUE}, {"X"=1043.0, "Y"=0.0, "Label"="Strip\t1043", "Coord On/Off"=TRUE}, {"X"=1044.0, "Y"=0.0, "Label"="Strip\t1044", "Coord On/Off"=TRUE}, {"X"=1045.0, "Y"=0.0, "Label"="Strip\t1045", "Coord On/Off"=TRUE}, {"X"=1046.0, "Y"=0.0, "Label"="Strip\t1046", "Coord On/Off"=TRUE}, {"X"=1047.0, "Y"=0.0, "Label"="Strip\t1047", "Coord On/Off"=TRUE}, {"X"=1048.0, "Y"=0.0, "Label"="Strip\t1048", "Coord On/Off"=TRUE}, {"X"=1049.0, "Y"=0.0, "Label"="Strip\t1049", "Coord On/Off"=TRUE}, {"X"=1050.0, "Y"=0.0, "Label"="Strip\t1050", "Coord On/Off"=TRUE}, {"X"=1051.0, "Y"=0.0, "Label"="Strip\t1051", "Coord On/Off"=TRUE}, {"X"=1052.0, "Y"=0.0, "Label"="Strip\t1052", "Coord On/Off"=TRUE}, {"X"=1053.0, "Y"=0.0, "Label"="Strip\t1053", "Coord On/Off"=TRUE}, {"X"=1054.0, "Y"=0.0, "Label"="Strip\t1054", "Coord On/Off"=TRUE}, {"X"=1055.0, "Y"=0.0, "Label"="Strip\t1055", "Coord On/Off"=TRUE}, {"X"=1056.0, "Y"=0.0, "Label"="Strip\t1056", "Coord On/Off"=TRUE}, {"X"=1057.0, "Y"=0.0, "Label"="Strip\t1057", "Coord On/Off"=TRUE}, {"X"=1058.0, "Y"=0.0, "Label"="Strip\t1058", "Coord On/Off"=TRUE}, {"X"=1059.0, "Y"=0.0, "Label"="Strip\t1059", "Coord On/Off"=TRUE}, {"X"=1060.0, "Y"=0.0, "Label"="Strip\t1060", "Coord On/Off"=TRUE}, {"X"=1061.0, "Y"=0.0, "Label"="Strip\t1061", "Coord On/Off"=TRUE}, {"X"=1062.0, "Y"=0.0, "Label"="Strip\t1062", "Coord On/Off"=TRUE}, {"X"=1063.0, "Y"=0.0, "Label"="Strip\t1063", "Coord On/Off"=TRUE}, {"X"=1064.0, "Y"=0.0, "Label"="Strip\t1064", "Coord On/Off"=TRUE}, {"X"=1065.0, "Y"=0.0, "Label"="Strip\t1065", "Coord On/Off"=TRUE}, {"X"=1066.0, "Y"=0.0, "Label"="Strip\t1066", "Coord On/Off"=TRUE}, {"X"=1067.0, "Y"=0.0, "Label"="Strip\t1067", "Coord On/Off"=TRUE}, {"X"=1068.0, "Y"=0.0, "Label"="Strip\t1068", "Coord On/Off"=TRUE}, {"X"=1069.0, "Y"=0.0, "Label"="Strip\t1069", "Coord On/Off"=TRUE}, {"X"=1070.0, "Y"=0.0, "Label"="Strip\t1070", "Coord On/Off"=TRUE}, {"X"=1071.0, "Y"=0.0, "Label"="Strip\t1071", "Coord On/Off"=TRUE}, {"X"=1072.0, "Y"=0.0, "Label"="Strip\t1072", "Coord On/Off"=TRUE}, {"X"=1073.0, "Y"=0.0, "Label"="Strip\t1073", "Coord On/Off"=TRUE}, {"X"=1074.0, "Y"=0.0, "Label"="Strip\t1074", "Coord On/Off"=TRUE}, {"X"=1075.0, "Y"=0.0, "Label"="Strip\t1075", "Coord On/Off"=TRUE}, {"X"=1076.0, "Y"=0.0, "Label"="Strip\t1076", "Coord On/Off"=TRUE}, {"X"=1077.0, "Y"=0.0, "Label"="Strip\t1077", "Coord On/Off"=TRUE}, {"X"=1078.0, "Y"=0.0, "Label"="Strip\t1078", "Coord On/Off"=TRUE}, {"X"=1079.0, "Y"=0.0, "Label"="Strip\t1079", "Coord On/Off"=TRUE}, {"X"=1080.0, "Y"=0.0, "Label"="Strip\t1080", "Coord On/Off"=TRUE}, {"X"=1081.0, "Y"=0.0, "Label"="Strip\t1081", "Coord On/Off"=TRUE}, {"X"=1082.0, "Y"=0.0, "Label"="Strip\t1082", "Coord On/Off"=TRUE}, {"X"=1083.0, "Y"=0.0, "Label"="Strip\t1083", "Coord On/Off"=TRUE}, {"X"=1084.0, "Y"=0.0, "Label"="Strip\t1084", "Coord On/Off"=TRUE}, {"X"=1085.0, "Y"=0.0, "Label"="Strip\t1085", "Coord On/Off"=TRUE}, {"X"=1086.0, "Y"=0.0, "Label"="Strip\t1086", "Coord On/Off"=TRUE}, {"X"=1087.0, "Y"=0.0, "Label"="Strip\t1087", "Coord On/Off"=TRUE}, {"X"=1088.0, "Y"=0.0, "Label"="Strip\t1088", "Coord On/Off"=TRUE}, {"X"=1089.0, "Y"=0.0, "Label"="Strip\t1089", "Coord On/Off"=TRUE}, {"X"=1090.0, "Y"=0.0, "Label"="Strip\t1090", "Coord On/Off"=TRUE}, {"X"=1091.0, "Y"=0.0, "Label"="Strip\t1091", "Coord On/Off"=TRUE}, {"X"=1092.0, "Y"=0.0, "Label"="Strip\t1092", "Coord On/Off"=TRUE}, {"X"=1093.0, "Y"=0.0, "Label"="Strip\t1093", "Coord On/Off"=TRUE}, {"X"=1094.0, "Y"=0.0, "Label"="Strip\t1094", "Coord On/Off"=TRUE}, {"X"=1095.0, "Y"=0.0, "Label"="Strip\t1095", "Coord On/Off"=TRUE}, {"X"=1096.0, "Y"=0.0, "Label"="Strip\t1096", "Coord On/Off"=TRUE}, {"X"=1097.0, "Y"=0.0, "Label"="Strip\t1097", "Coord On/Off"=TRUE}, {"X"=1098.0, "Y"=0.0, "Label"="Strip\t1098", "Coord On/Off"=TRUE}, {"X"=1099.0, "Y"=0.0, "Label"="Strip\t1099", "Coord On/Off"=TRUE}, {"X"=1100.0, "Y"=0.0, "Label"="Strip\t1100", "Coord On/Off"=TRUE}, {"X"=1101.0, "Y"=0.0, "Label"="Strip\t1101", "Coord On/Off"=TRUE}, {"X"=1102.0, "Y"=0.0, "Label"="Strip\t1102", "Coord On/Off"=TRUE}, {"X"=1103.0, "Y"=0.0, "Label"="Strip\t1103", "Coord On/Off"=TRUE}, {"X"=1104.0, "Y"=0.0, "Label"="Strip\t1104", "Coord On/Off"=TRUE}, {"X"=1105.0, "Y"=0.0, "Label"="Strip\t1105", "Coord On/Off"=TRUE}, {"X"=1106.0, "Y"=0.0, "Label"="Strip\t1106", "Coord On/Off"=TRUE}, {"X"=1107.0, "Y"=0.0, "Label"="Strip\t1107", "Coord On/Off"=TRUE}, {"X"=1108.0, "Y"=0.0, "Label"="Strip\t1108", "Coord On/Off"=TRUE}, {"X"=1109.0, "Y"=0.0, "Label"="Strip\t1109", "Coord On/Off"=TRUE}, {"X"=1110.0, "Y"=0.0, "Label"="Strip\t1110", "Coord On/Off"=TRUE}, {"X"=1111.0, "Y"=0.0, "Label"="Strip\t1111", "Coord On/Off"=TRUE}, {"X"=1112.0, "Y"=0.0, "Label"="Strip\t1112", "Coord On/Off"=TRUE}, {"X"=1113.0, "Y"=0.0, "Label"="Strip\t1113", "Coord On/Off"=TRUE}, {"X"=1114.0, "Y"=0.0, "Label"="Strip\t1114", "Coord On/Off"=TRUE}, {"X"=1115.0, "Y"=0.0, "Label"="Strip\t1115", "Coord On/Off"=TRUE}, {"X"=1116.0, "Y"=0.0, "Label"="Strip\t1116", "Coord On/Off"=TRUE}, {"X"=1117.0, "Y"=0.0, "Label"="Strip\t1117", "Coord On/Off"=TRUE}, {"X"=1118.0, "Y"=0.0, "Label"="Strip\t1118", "Coord On/Off"=TRUE}, {"X"=1119.0, "Y"=0.0, "Label"="Strip\t1119", "Coord On/Off"=TRUE}, {"X"=1120.0, "Y"=0.0, "Label"="Strip\t1120", "Coord On/Off"=TRUE}, {"X"=1121.0, "Y"=0.0, "Label"="Strip\t1121", "Coord On/Off"=TRUE}, {"X"=1122.0, "Y"=0.0, "Label"="Strip\t1122", "Coord On/Off"=TRUE}, {"X"=1123.0, "Y"=0.0, "Label"="Strip\t1123", "Coord On/Off"=TRUE}, {"X"=1124.0, "Y"=0.0, "Label"="Strip\t1124", "Coord On/Off"=TRUE}, {"X"=1125.0, "Y"=0.0, "Label"="Strip\t1125", "Coord On/Off"=TRUE}, {"X"=1126.0, "Y"=0.0, "Label"="Strip\t1126", "Coord On/Off"=TRUE}, {"X"=1127.0, "Y"=0.0, "Label"="Strip\t1127", "Coord On/Off"=TRUE}, {"X"=1128.0, "Y"=0.0, "Label"="Strip\t1128", "Coord On/Off"=TRUE}, {"X"=1129.0, "Y"=0.0, "Label"="Strip\t1129", "Coord On/Off"=TRUE}, {"X"=1130.0, "Y"=0.0, "Label"="Strip\t1130", "Coord On/Off"=TRUE}, {"X"=1131.0, "Y"=0.0, "Label"="Strip\t1131", "Coord On/Off"=TRUE}, {"X"=1132.0, "Y"=0.0, "Label"="Strip\t1132", "Coord On/Off"=TRUE}, {"X"=1133.0, "Y"=0.0, "Label"="Strip\t1133", "Coord On/Off"=TRUE}, {"X"=1134.0, "Y"=0.0, "Label"="Strip\t1134", "Coord On/Off"=TRUE}, {"X"=1135.0, "Y"=0.0, "Label"="Strip\t1135", "Coord On/Off"=TRUE}, {"X"=1136.0, "Y"=0.0, "Label"="Strip\t1136", "Coord On/Off"=TRUE}, {"X"=1137.0, "Y"=0.0, "Label"="Strip\t1137", "Coord On/Off"=TRUE}, {"X"=1138.0, "Y"=0.0, "Label"="Strip\t1138", "Coord On/Off"=TRUE}, {"X"=1139.0, "Y"=0.0, "Label"="Strip\t1139", "Coord On/Off"=TRUE}, {"X"=1140.0, "Y"=0.0, "Label"="Strip\t1140", "Coord On/Off"=TRUE}, {"X"=1141.0, "Y"=0.0, "Label"="Strip\t1141", "Coord On/Off"=TRUE}, {"X"=1142.0, "Y"=0.0, "Label"="Strip\t1142", "Coord On/Off"=TRUE}, {"X"=1143.0, "Y"=0.0, "Label"="Strip\t1143", "Coord On/Off"=TRUE}, {"X"=1144.0, "Y"=0.0, "Label"="Strip\t1144", "Coord On/Off"=TRUE}, {"X"=1145.0, "Y"=0.0, "Label"="Strip\t1145", "Coord On/Off"=TRUE}, {"X"=1146.0, "Y"=0.0, "Label"="Strip\t1146", "Coord On/Off"=TRUE}, {"X"=1147.0, "Y"=0.0, "Label"="Strip\t1147", "Coord On/Off"=TRUE}, {"X"=1148.0, "Y"=0.0, "Label"="Strip\t1148", "Coord On/Off"=TRUE}, {"X"=1149.0, "Y"=0.0, "Label"="Strip\t1149", "Coord On/Off"=TRUE}, {"X"=1150.0, "Y"=0.0, "Label"="Strip\t1150", "Coord On/Off"=TRUE}, {"X"=1151.0, "Y"=0.0, "Label"="Strip\t1151", "Coord On/Off"=TRUE}, {"X"=1152.0, "Y"=0.0, "Label"="Strip\t1152", "Coord On/Off"=TRUE}, {"X"=1153.0, "Y"=0.0, "Label"="Strip\t1153", "Coord On/Off"=TRUE}, {"X"=1154.0, "Y"=0.0, "Label"="Strip\t1154", "Coord On/Off"=TRUE}]}, ...(4 in all)])   [LabVIEW 2018]
doc: "Utility to read probe plan from text file and generate respective coordinates in global variable."
uses:
  general_VIs/globals/QC_MeasurementSetup.vi
  ProbePlanParams.vi
  <vilib>/regexp/Match Regular Expression.xnode
panel:
  out "Last Index":i32=4361
  out "No. probe points":string="1026 probe points"
  in  "ProbePoints":T2
